vi "ExtractRobotPosition.vi"(8 "DistanceThresh":sgl, 9 "MarkerIdx":i32=4, 10 "BodyIdx":i32=4, 11 "Data":string) -> (1 "Found?":bool, 2 "RigidBodyOri":sgl[](array[numeric]), 3 "RigidBodyPos":sgl[](array[numeric]))   [LabVIEW 2011]
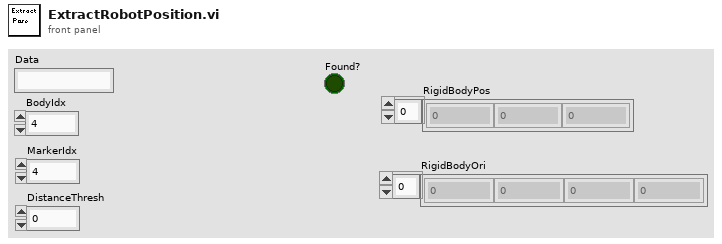
[diagram p1: front panel]
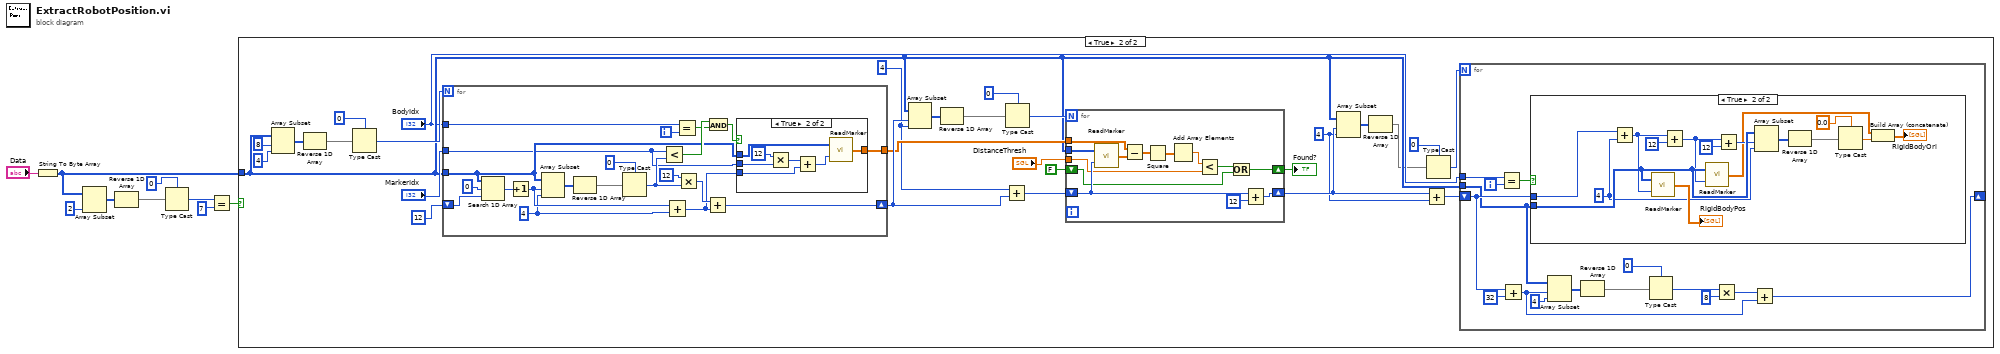
[diagram p0: block diagram]
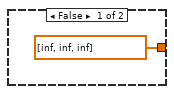
[diagram p4: hidden frame]
diagram:
  n1 = String To Byte Array(string="Data") -> (unsigned byte array=w3:u8[])
  n2 = Array Subset(array=w3, length=2) -> (w2:u8[])  [unwired: 1 in]
  n3 = Reverse 1D Array(array=w2) -> (reversed array=w1:u8[])
  n4 = Type Cast(type=i16 0, x=w1) -> (*(type *) &x=w6:i16)
  n5 = Equal?(x=w6, y=i16 7) -> (x = y?=w4:bool)
  n6 = case shown="True" w4 {
    tunnel: w3 -> [_ w18]
    frame False {
    }
    frame True {
      w13 = 4 ("y")
      w15 = 4 ("length")
      n7 = Array Subset(array=w18, index=8, length=4) -> (w35:u8[])
      n8 = Reverse 1D Array(array=w35) -> (reversed array=w12:u8[])
      n9 = Type Cast(type=0, x=w12) -> (*(type *) &x=w32:i32)
      n10 = for {
        N: w32 -> [_]
        shift-right: [w81] -> w27
        shift-left: 12 -> [w100]
        tunnel: w18 -> [w89]
        tunnel: "BodyIdx" -> [w95]
        tunnel: "MarkerIdx" -> [w88]
        tunnel: [w87] -> w25
        i -> [w94]
        w84 = 4 ("length")
        n11 = Search 1D Array(1D array=w89, element=u8 0, start index (0)=w100) -> (index of element=w97:i32)
        n12 = Increment(x=w97) -> (x+1=w85:i32)
        n13 = Array Subset(array=w89, index=w85, length=w84) -> (w98:u8[])
        n14 = Reverse 1D Array(array=w98) -> (reversed array=w86:u8[])
        n15 = Type Cast(type=0, x=w86) -> (*(type *) &x=w93:i32)
        n16 = Less?(x=w88, y=w93) -> (x < y?=w92:bool)
        n17 = Add(x=w85, y=w84) -> (x+y=w82:i32)
        n18 = Equal?(x=w95, y=w94) -> (x = y?=w91:bool)
        n19 = Multiply(x=12, y=w93) -> (x*y=w83:i32)
        n20 = Add(x=w83, y=w82) -> (x+y=w81:i32)
        n21 = And(x=w92, y=w91) -> (x .and. y?=w90:bool)
        n22 = case shown="True" w90 {
          tunnel: w89 -> [_ w109]
          tunnel: w88 -> [_ w104]
          tunnel: [sgl[] [inf, inf, inf] w108] -> w87
          tunnel: w82 -> [_ w107]
          frame False {
          }
          frame True {
            n23 = Multiply(x=12, y=w104) -> (x*y=w103:i32)
            n24 = Add(x=w103, y=w107) -> (x+y=w106:i32)
            n25 = call "ReadMarker.vi"("MarkerIdx"=w106, "Data"=w109) -> ("Marker"=w108:sgl[])
          }
        }
      }
      n26 = Array Subset(array=w18, index=w27, length=w15) -> (w29:u8[])
      n27 = Reverse 1D Array(array=w29) -> (reversed array=w11:u8[])
      n28 = Add(x=w15, y=w27) -> (x+y=w26:i32)
      n29 = Type Cast(type=0, x=w11) -> (*(type *) &x=w28:i32)
      n30 = for {
        N: w28 -> [_]
        shift-right: [w78] -> w16
        shift-left: w26 -> [w77]
        tunnel: w18 -> [w80]
        tunnel: w25 -> [w76]
        shift-right: [w69] -> w23
        shift-left: FALSE -> [w70]
        tunnel: "DistanceThresh" -> [w68]
        n31 = call "ReadMarker.vi"("MarkerIdx"=w77, "Data"=w80) -> ("Marker"=w75:sgl[])
        n32 = Subtract(x=w76, y=w75) -> (x-y=w74:sgl[])
        n33 = Square(x=w74) -> (x^2=w73:sgl[])
        n34 = Add Array Elements(numeric array=w73) -> (sum=w71:sgl)
        n35 = Less?(x=w71, y=w68) -> (x < y?=w72:bool)
        n36 = Or(x=w72, y=w70) -> (x .or. y?=w69:bool)
        n37 = Add(x=w77, y=12) -> (x+y=w78:i32)
      }
      "Found?" <- w23
      n38 = Array Subset(array=w18, index=w16, length=w13) -> (w20:u8[])
      n39 = Reverse 1D Array(array=w20) -> (reversed array=w10:u8[])
      n40 = Add(x=w16, y=w13) -> (x+y=w21:i32)
      n41 = Type Cast(type=0, x=w10) -> (*(type *) &x=w17:i32)
      n42 = for {
        N: w17 -> [_]
        tunnel: w18 -> [w47]
        tunnel: "BodyIdx" -> [w52]
        shift-right: [w39] -> _
        shift-left: w21 -> [w49]
        i -> [w51]
        n43 = Equal?(x=w52, y=w51) -> (x = y?=w50:bool)
        n44 = Add(x=w49, y=32) -> (x+y=w40:i32)
        n45 = case shown="True" w50 {
          tunnel: w47 -> [_ w63]
          tunnel: w49 -> [_ w65]
          frame False {
          }
          frame True {
            w59 = 4 ("y")
            n46 = Add(x=w65, y=w59) -> (x+y=w64:i32)
            n47 = call "ReadMarker.vi"("MarkerIdx"=w64, "Data"=w63) -> ("Marker"=→"RigidBodyPos":sgl[])
            n48 = Add(x=w64, y=12) -> (x+y=w61:i32)
            n49 = call "ReadMarker.vi"("MarkerIdx"=w61, "Data"=w63) -> ("Marker"=w55:sgl[])
            n50 = Add(x=w61, y=12) -> (x+y=w60:i32)
            n51 = Array Subset(array=w63, index=w60, length=w59) -> (w58:u8[])
            n52 = Reverse 1D Array(array=w58) -> (reversed array=w56:u8[])
            n53 = Type Cast(type=sgl 0.0, x=w56) -> (*(type *) &x=w54:sgl)
            n54 = Build Array (concatenate)(w55, w54) -> (→"RigidBodyOri":sgl[])
          }
        }
        n55 = Array Subset(array=w47, index=w40, length=4) -> (w44:u8[])
        n56 = Reverse 1D Array(array=w44) -> (reversed array=w38:u8[])
        n57 = Type Cast(type=0, x=w38) -> (*(type *) &x=w43:i32)
        n58 = Multiply(x=w43, y=8) -> (x*y=w41:i32)
        n59 = Add(x=w41, y=w40) -> (x+y=w39:i32)
      }
    }
  }
